vi "File_In_Use.vi"(7 "Action":T1, 8 "Error In":errorcluster, 11 "Path IN":path) -> (0 "Error Out":errorcluster, 1 "File/Folder not found":bool, 2 "Cancelled?":bool, 3 "Path OUT":path)   [LabVIEW 2012]
doc: "SciScan 1.2 160622\nThis VI lets the user to close any resources that may be open while attempting to write/delete"
uses:
  File_In_Use__Commands.ctl
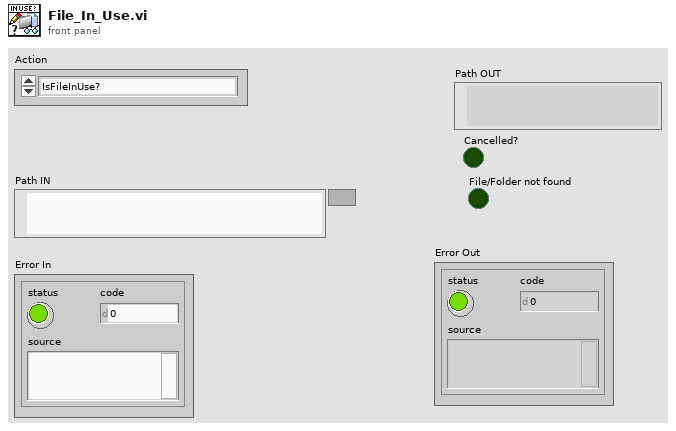
[diagram p1: front panel]
types:
  T1 = typedef "File_In_Use__Commands.ctl" = enum16{"IsFileInUse?", "IsFolderInUse?"}
  T2 = enum16{"open", "replace", "create", "open or create", "replace or create", "replace or create with confirmation"}
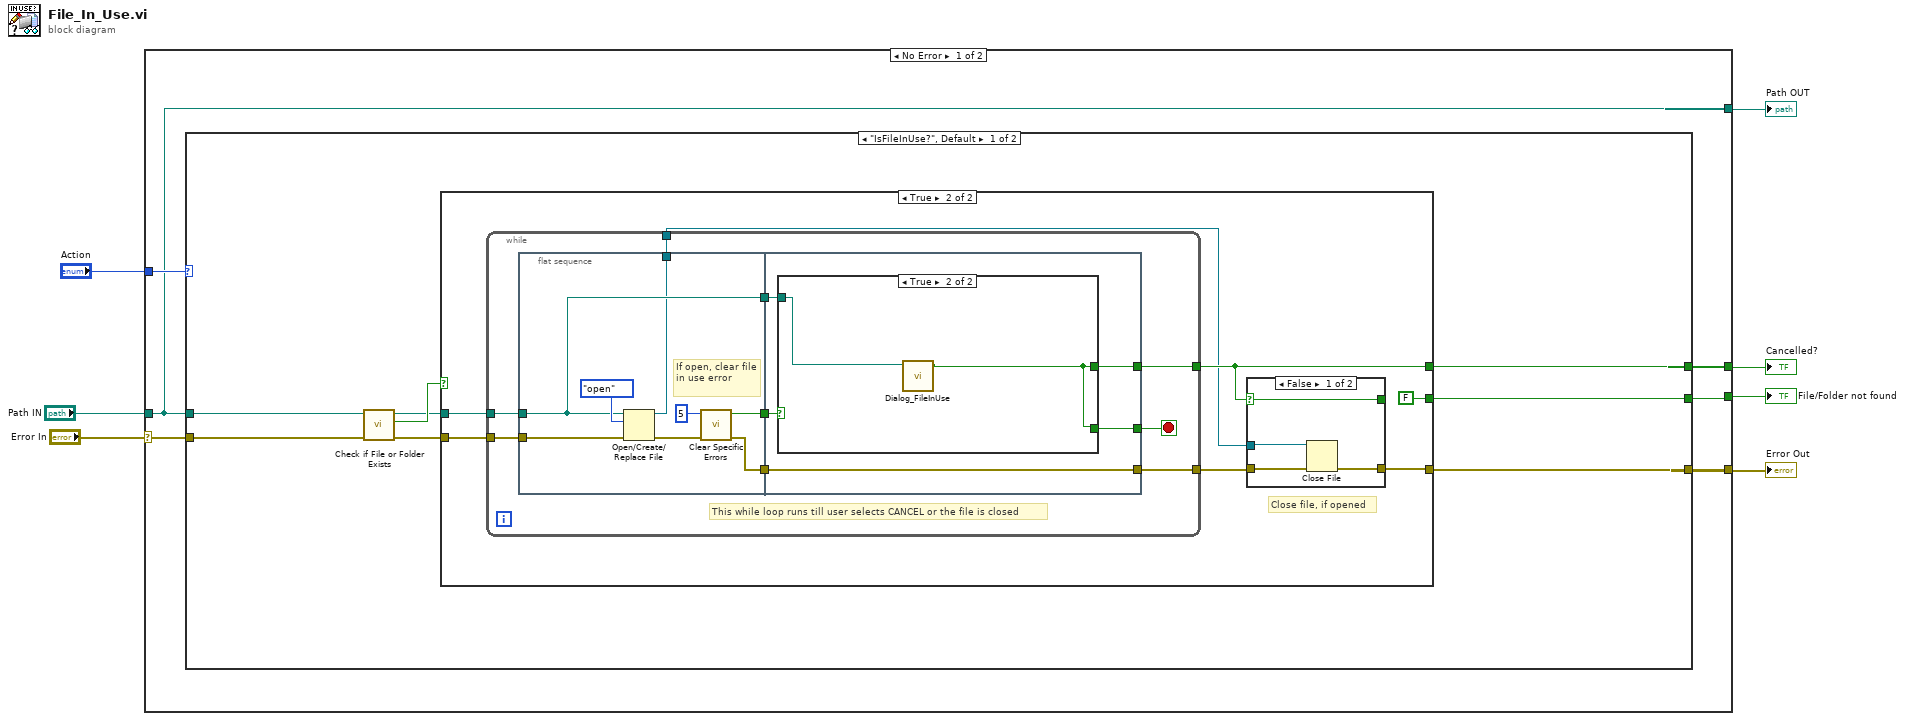
[diagram p0: block diagram]
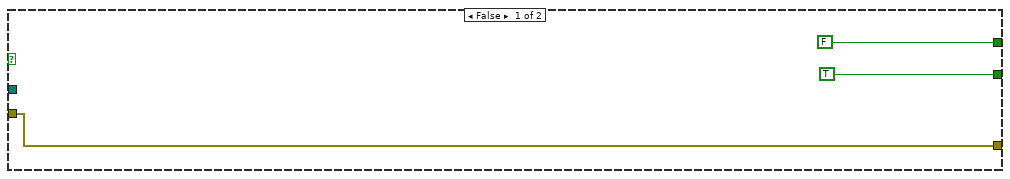
[diagram p2: hidden frame]
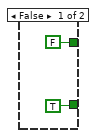
[diagram p4: hidden frame]
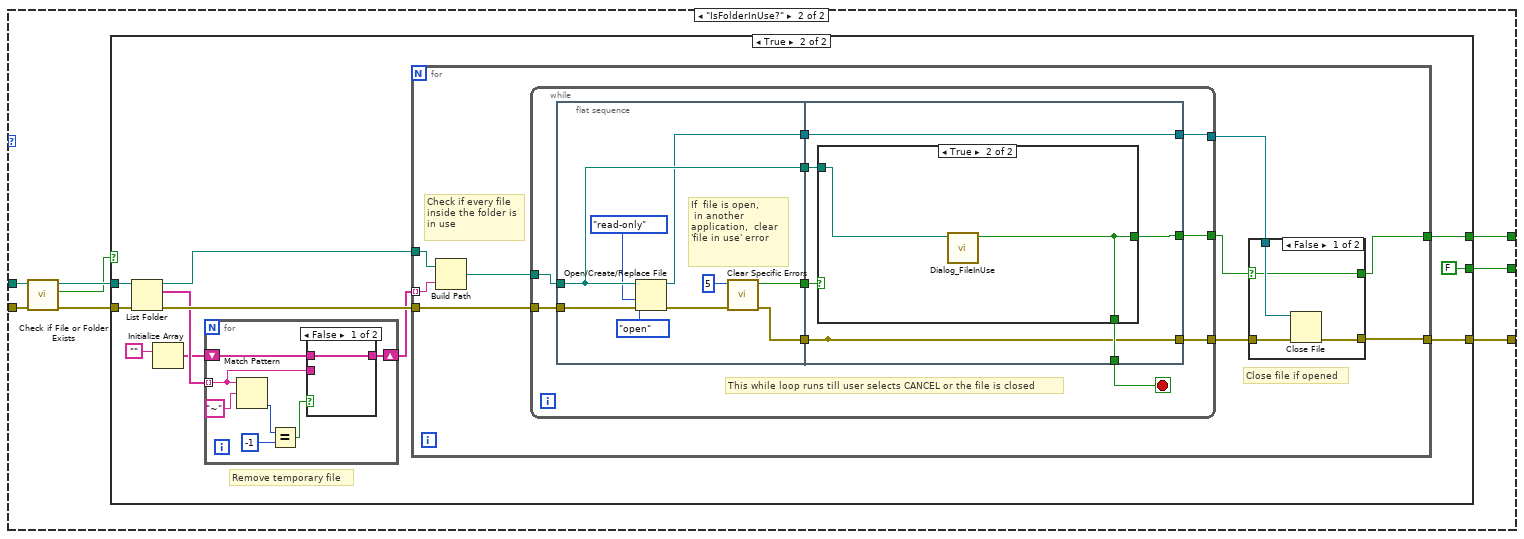
[diagram p5: hidden frame]
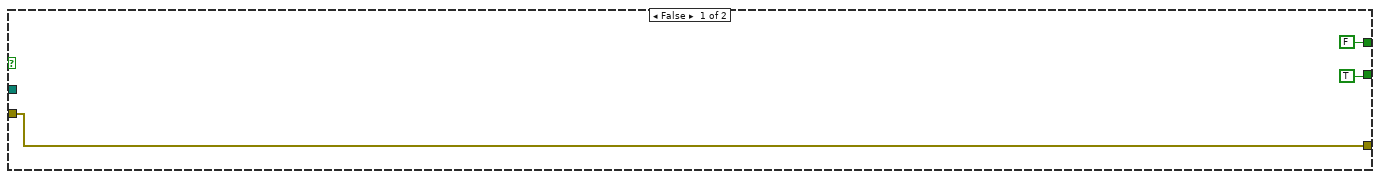
[diagram p6: hidden frame]
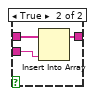
[diagram p7: hidden frame]
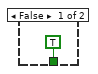
[diagram p9: hidden frame]
diagram:
  n1 = case shown="No Error" "Error In" {
    selector: "Error In" -> [w11 w141]
    tunnel: "Path IN" -> [w9 w140]
    tunnel: [w13 w141] -> w6
    tunnel: "Action" -> [w12 _]
    tunnel: [w10 _] -> w3
    tunnel: [w9 w140] -> w2
    tunnel: [w8 _] -> w1
    frame No Error {
      n2 = case shown="\"IsFileInUse?\", Default" w12 {
        tunnel: w9 -> [w18 w68]
        tunnel: [w21 w71] -> w13
        tunnel: w11 -> [w19 w69]
        tunnel: [w20 w70] -> w10
        tunnel: [w14 w64] -> w8
        frame "IsFileInUse?", Default {
          n3 = call <vilib>:"Check if File or Folder Exists.vi"("error in (no error)"=w19, "path"=w18) -> ("error out"=w17:errorcluster, "file or folder exists?"=w16:bool, "dup path"=w15:path)  [unwired: 7 in]
          n4 = case shown="True" w16 {
            tunnel: [w24 w27] -> w21
            tunnel: [FALSE ("T button?") w26] -> w20
            tunnel: w17 -> [w24 w31]
            tunnel: w15 -> [_ w30]
            tunnel: [TRUE ("T button?") FALSE ("T button?")] -> w14
            frame False {
            }
            frame True {
              # "Close file, if opened"
              n5 = while {
                tunnel: w30 -> [w39]
                tunnel: [w43] -> w28
                tunnel: w31 -> [w40]
                tunnel: [w41] -> w26
                tunnel: [w38] -> w25
                stop <- w44 stop-if-true
                # "This while loop runs till user selects CANCEL or the file is closed"
                n6 = flat-sequence {
                  tunnel: w39 -> [w49]
                  tunnel: [w51] -> w46
                  tunnel: [w50] -> w45
                  tunnel: [w49] -> w42
                  tunnel: w40 -> [w48]
                  tunnel: [w47] -> w38
                  tunnel: w46 -> [w59]
                  tunnel: w45 -> [w58]
                  tunnel: [w58] -> w43
                  tunnel: [w57] -> w44
                  tunnel: w42 -> [w56]
                  tunnel: [w55] -> w41
                  frame #0 {
                    # "If open, clear file in use error"
                    n7 = Open/Create/Replace File(file path (use dialog)=w49, error in=w48, operation (0:open)=T2."open") -> (refnum out=w47:refnum<file>, error out=w52:errorcluster)  [unwired: 3 in, 1 out]
                    n8 = call "Clear Specific Errors.vi"("Error In"=w52, "Error number In"=5) -> ("Error Out"=w50:errorcluster, "Error Cleared?"=w51:bool)  [unwired: 8 in]
                  }
                  frame #1 {
                    n9 = case shown="True" w59 {
                      tunnel: [TRUE ("T button?") w62] -> w57
                      tunnel: w56 -> [_ w63]
                      tunnel: [FALSE ("T button?") w62] -> w55
                      frame False {
                      }
                      frame True {
                        n10 = call "Dialog_FileInUse.vi"("Path"=w63) -> ("Cancelled"=w62:bool)  [unwired: 10 in]
                      }
                    }
                  }
                }
              }
              n11 = case shown="False" w26 {
                selector: w26 -> [w32 w37]
                tunnel: w28 -> [w35 w36]
                tunnel: [w34 w36] -> w27
                tunnel: w25 -> [w33 _]
                tunnel: [w32 w37] -> _
                frame False {
                  n12 = Close File(refnum=w33, error in=w35) -> (error out=w34:errorcluster)  [unwired: 1 out]
                }
                frame True {
                }
              }
            }
          }
        }
        frame "IsFolderInUse?" {
          n13 = call <vilib>:"Check if File or Folder Exists.vi"("error in (no error)"=w69, "path"=w68) -> ("error out"=w66:errorcluster, "file or folder exists?"=w65:bool, "dup path"=w67:path)  [unwired: 7 in]
          n14 = case shown="True" w65 {
            tunnel: [w72 w85] -> w71
            tunnel: [FALSE w84] -> w70
            tunnel: w66 -> [w72 w83]
            tunnel: w67 -> [_ w82]
            tunnel: [TRUE FALSE] -> w64
            frame False {
            }
            frame True {
              # "Remove temporary file"
              n15 = List Folder(path=w82, error in=w83) -> (path out=w80:path, filenames=w79:string[], error out=w81:errorcluster)  [unwired: 2 in, 1 out]
              n16 = Initialize Array("") -> (w77:string[])  [unwired: 1 in]
              n17 = for {
                tunnel: w79 -> [w87] mode=indexing
                shift-right: [w86] -> w76
                shift-left: w77 -> [w91]
                n18 = Match Pattern(string=w87, regular expression="~") -> (offset past match=w90:i32)  [unwired: 1 in, 3 out]
                n19 = Equal?(x=w90, y=-1) -> (x = y?=w88:bool)
                n20 = case shown="False" w88 {
                  tunnel: w91 -> [w93 w96]
                  tunnel: w87 -> [_ w95]
                  tunnel: [w93 w94] -> w86
                  frame False {
                  }
                  frame True {
                    n21 = Insert Into Array(array=w96, new element=w95) -> (w94:string[])  [unwired: 1 in]
                  }
                }
              }
              n22 = for {
                tunnel: [w97] -> w85
                tunnel: [w98] -> w84
                tunnel: w81 -> [w103]
                tunnel: w76 -> [w104] mode=indexing
                tunnel: w80 -> [w105]
                # "Close file if opened"
                # "Check if every file \ninside the folder is\nin use"
                n23 = Build Path(base path=w105, name or relative path=w104) -> (appended path=w102:path)
                n24 = while {
                  tunnel: w102 -> [w121]
                  tunnel: w103 -> [w116]
                  tunnel: [w114] -> w100
                  tunnel: [w113] -> w101
                  tunnel: [w112] -> w99
                  stop <- w118 stop-if-true
                  # "This while loop runs till user selects CANCEL or the file is closed"
                  n25 = flat-sequence {
                    tunnel: w121 -> [w125]
                    tunnel: [w129] -> w120
                    tunnel: [w128] -> w119
                    tunnel: [w125] -> w117
                    tunnel: w116 -> [w127]
                    tunnel: [w124] -> w115
                    tunnel: w120 -> [w136]
                    tunnel: w119 -> [w131]
                    tunnel: [w135] -> w118
                    tunnel: w117 -> [w134]
                    tunnel: w115 -> [w133]
                    tunnel: [w133] -> w112
                    tunnel: [w131] -> _
                    tunnel: [w132] -> w114
                    tunnel: [w131] -> w113
                    frame #0 {
                      # "If  file is open,\n in another application,  clear 'file in use' error"
                      n26 = Open/Create/Replace File(file path (use dialog)=w125, error in=w127, operation (0:open)=T2."open", access (0:read/write)=enum16{"read/write", "read-only", "write-only"}."read-only") -> (refnum out=w124:refnum<file>, error out=w126:errorcluster)  [unwired: 2 in, 1 out]
                      n27 = call "Clear Specific Errors.vi"("Error In"=w126, "Error number In"=5) -> ("Error Out"=w128:errorcluster, "Error Cleared?"=w129:bool)  [unwired: 8 in]
                    }
                    frame #1 {
                      n28 = case shown="True" w136 {
                        tunnel: [TRUE ("T button?") w138] -> w135
                        tunnel: w134 -> [_ w139]
                        tunnel: [_ w138] -> w132
                        frame False {
                        }
                        frame True {
                          n29 = call "Dialog_FileInUse.vi"("Path"=w139) -> ("Cancelled"=w138:bool)  [unwired: 10 in]
                        }
                      }
                    }
                  }
                }
                n30 = case shown="False" w100 {
                  selector: w100 -> [w106 w111]
                  tunnel: w101 -> [w109 w110]
                  tunnel: [w108 w110] -> w97
                  tunnel: w99 -> [w107 _]
                  tunnel: [w106 w111] -> w98
                  frame False {
                    n31 = Close File(refnum=w107, error in=w109) -> (error out=w108:errorcluster)  [unwired: 1 out]
                  }
                  frame True {
                  }
                }
              }
            }
          }
        }
      }
    }
    frame Error {
    }
  }
  "Error Out" <- w6
  "Cancelled?" <- w3
  "Path OUT" <- w2
  "File/Folder not found" <- w1
